vi "S_absolu.vi"(10 "Th  (Seebeck)":u16(ring)=5 items=["B", "E", "J", "K", "R", "S", "T", "N"], 11 "T, in  Kelvin":dbl) -> (1 "TC signal /microVperK":dbl, 2 "S of - wire /microV/K":dbl, 3 "S of + wire /microV/K":dbl)   [LabVIEW 2018]
panel:
  in  "error in":errorcluster
  out "error out":errorcluster
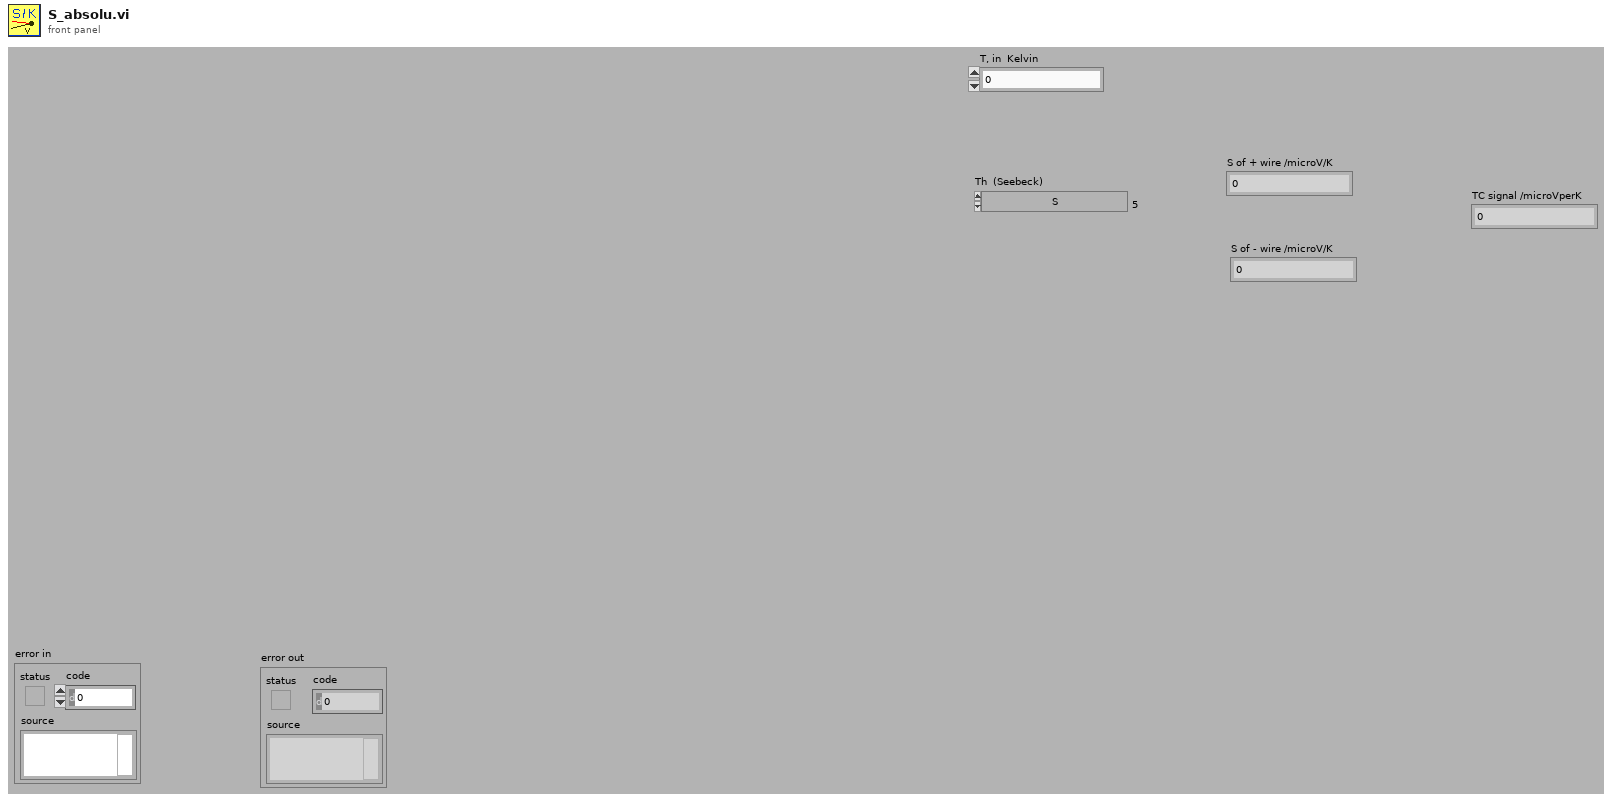
[diagram p1: front panel]
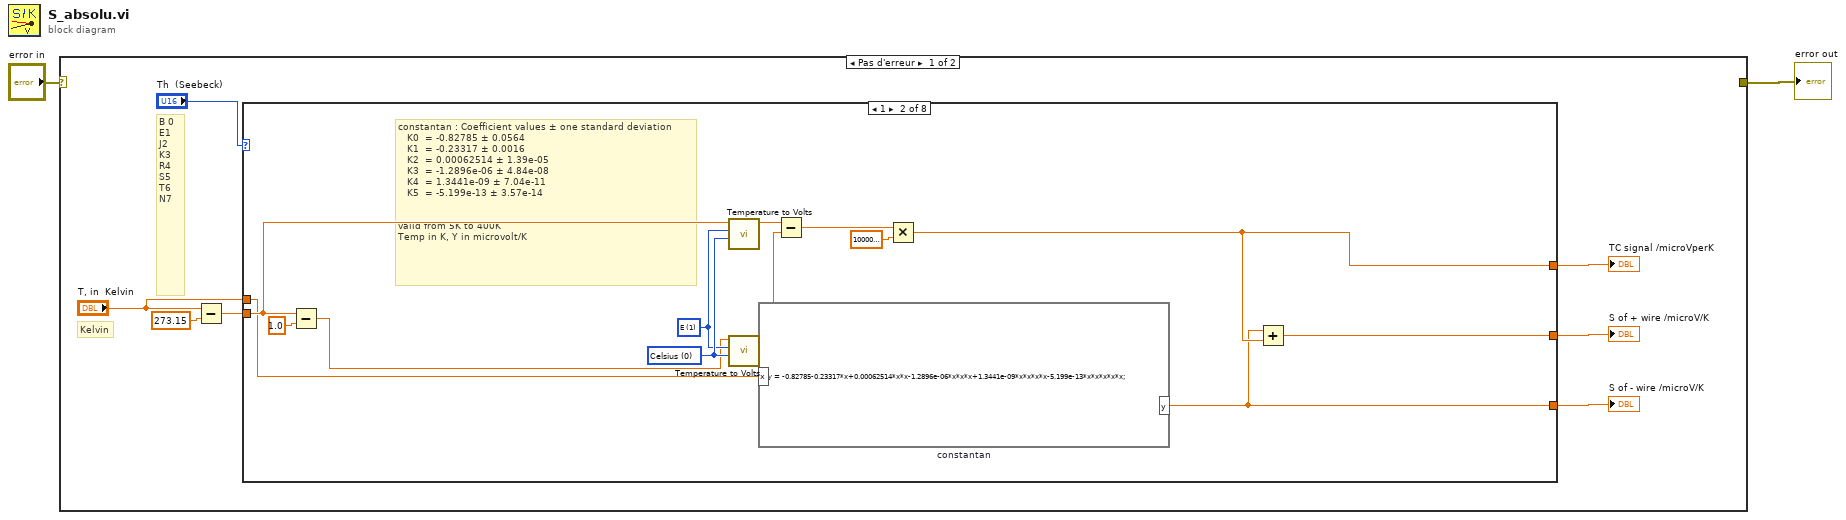
[diagram p0: block diagram]
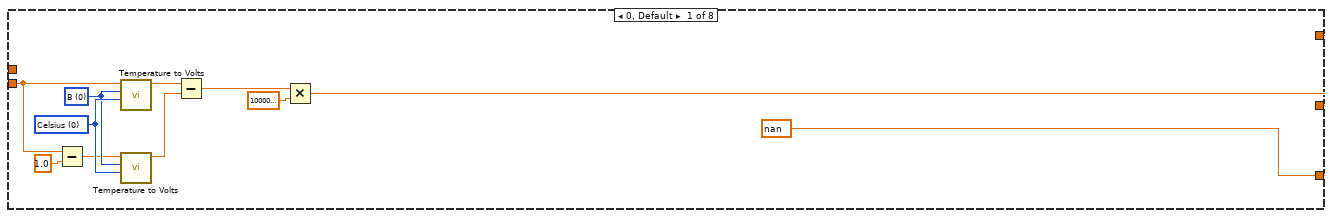
[diagram p2: hidden frame]
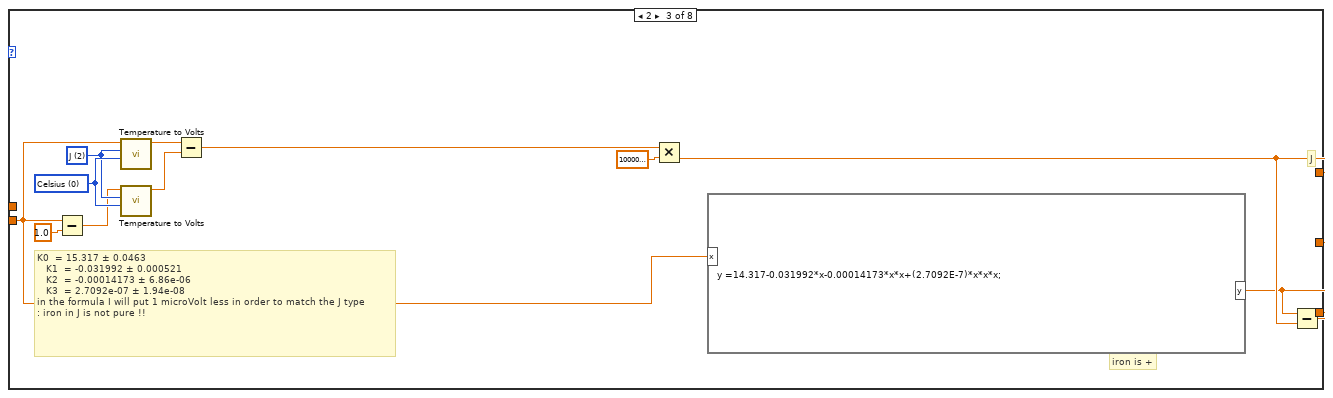
[diagram p3: hidden frame]
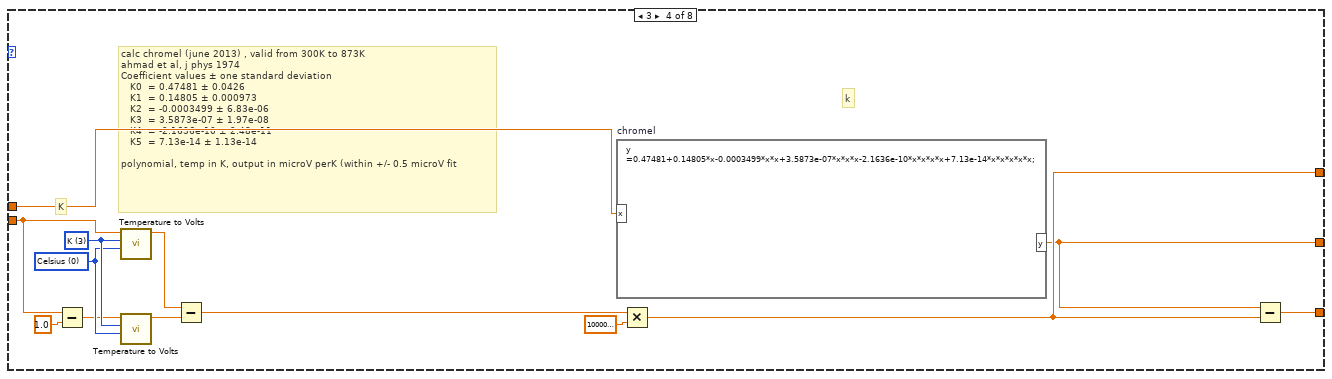
[diagram p4: hidden frame]
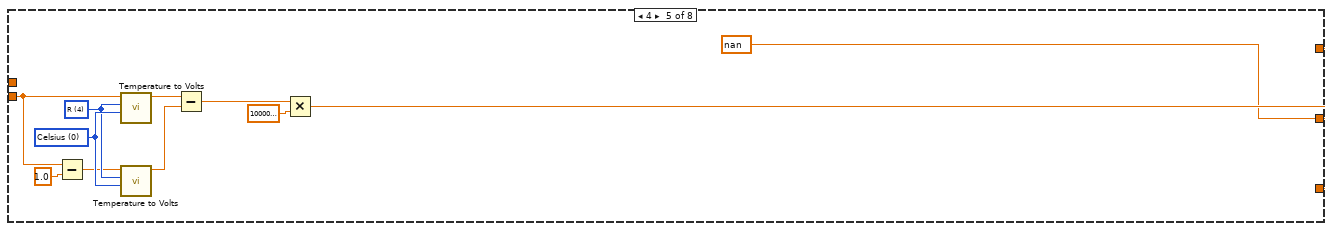
[diagram p5: hidden frame]
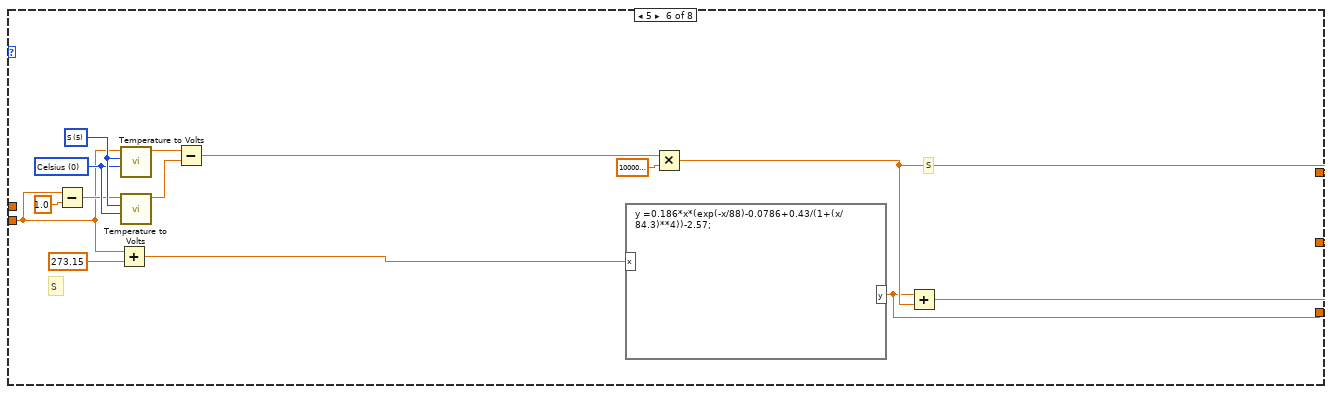
[diagram p6: hidden frame]
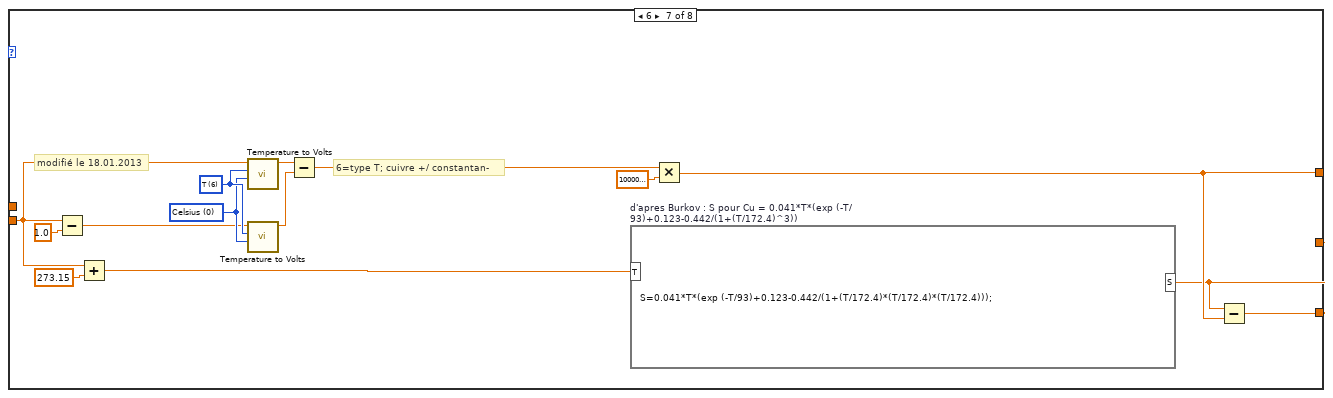
[diagram p7: hidden frame]
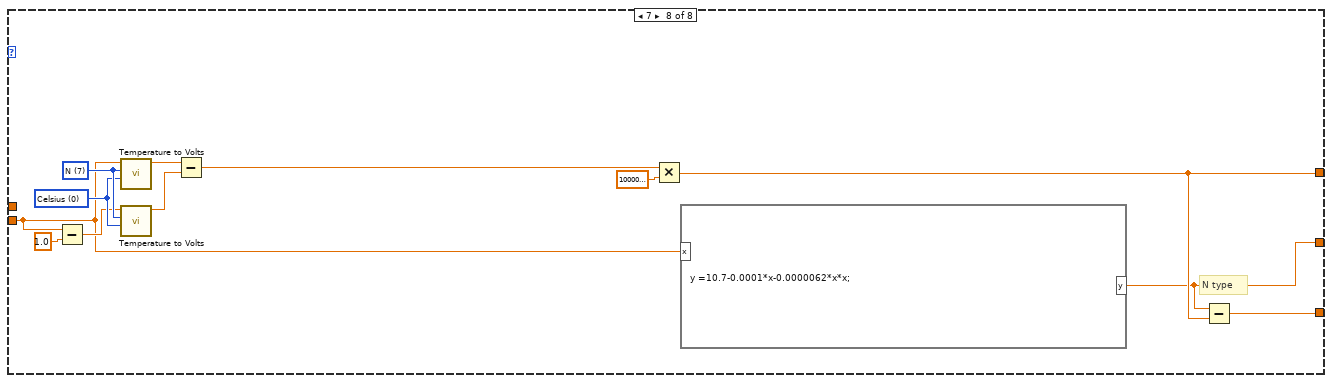
[diagram p8: hidden frame]
diagram:
  n1 = case shown="Pas d'erreur" "error in" {
    selector: "error in" -> [_ w110]
    tunnel: [_ w110] -> w2
    frame No Error {
      # "Kelvin"
      # "B 0\nE1\nJ2\nK3\nR4\nS5\nT6\nN7"
      n2 = Subtract(x="T, in  Kelvin", y=273.15) -> (x-y=w4:dbl)
      n3 = case shown="1" "Th  (Seebeck)" {
        tunnel: [w20 w22 w34 w58 w59 w70 w89 w101] -> w8
        tunnel: w4 -> [w10 w24 w37 w48 w61 w73 w85 w98]
        tunnel: [w20 w21 w35 w47 w59 w75 w84 w99] -> w6
        tunnel: [w11 w25 w36 w49 w60 w74 w88 w100] -> w7
        tunnel: "T, in  Kelvin" -> [_ w23 _ w46 _ _ _ _]
        frame 0, Default {
          w17 = u16 0 items=["B", "E", "J", "K", "R", "S", "T", "N"] ("ThermocoupleType")
          w19 = u16 0 items=["Celsius", "Fahrenheit", "Kelvin", "Rankine"] ("Temperature Units")
          w20 = nan
          n4 = Subtract(x=w10, y=1.0) -> (x-y=w15:dbl)
          n5 = call <vilib>:"Temperature to Volts.vi"("Temperature Units"=w19, "ThermocoupleType"=w17, "Temperature"=w10) -> ("Thermocouple Voltage"=w14:sgl)  [unwired: 4 out]
          n6 = call <vilib>:"Temperature to Volts.vi"("Temperature Units"=w19, "ThermocoupleType"=w17, "Temperature"=w15) -> ("Thermocouple Voltage"=w13:sgl)  [unwired: 4 out]
          n7 = Subtract(x=w14, y=w13) -> (x-y=w12:sgl)
          n8 = Multiply(x=w12, y=1000000.0) -> (x*y=w11:dbl)
        }
        frame 1 {
          w31 = u16 1 items=["B", "E", "J", "K", "R", "S", "T", "N"] ("ThermocoupleType")
          w33 = u16 0 items=["Celsius", "Fahrenheit", "Kelvin", "Rankine"] ("Temperature Units")
          # "constantan : Coefficient values ± one standard deviation\n  \tK0 \t= -0.82785 ± 0.0564\n  \tK1 \t= -0.23317 ± 0.0016\n  \tK2 \t= 0.00062514 ± 1.39e-05\n  \tK3 \t= -1.2896e-06 ± 4.84e-08\n  \tK4 \t= 1.3441e-09 ± 7.04e-11\n  \tK5 \t= -5.199e-13 ± 3.57e-14\n\n\nvalid from 5K to 400K\nTemp in K, Y in microvolt/K"
          n9 = Subtract(x=w24, y=1.0) -> (x-y=w29:dbl)
          n10 = call <vilib>:"Temperature to Volts.vi"("Temperature Units"=w33, "ThermocoupleType"=w31, "Temperature"=w24) -> ("Thermocouple Voltage"=w28:sgl)  [unwired: 4 out]
          n11 = call <vilib>:"Temperature to Volts.vi"("Temperature Units"=w33, "ThermocoupleType"=w31, "Temperature"=w29) -> ("Thermocouple Voltage"=w27:sgl)  [unwired: 4 out]
          n12 = formula code="y = -0.82785-0.23317*x+0.00062514*x*x-1.2896e-06*x*x*x+1.3441e-09*x*x*x*x-5.199e-13*x*x*x*x*x;" "constantan"("x"=w23) -> ("y"=w22:dbl)
          n13 = Subtract(x=w28, y=w27) -> (x-y=w26:sgl)
          n14 = Multiply(x=w26, y=1000000.0) -> (x*y=w25:dbl)
          n15 = Add(x=w22, y=w25) -> (x+y=w21:dbl)
        }
        frame 2 {
          w43 = u16 2 items=["B", "E", "J", "K", "R", "S", "T", "N"] ("ThermocoupleType")
          w45 = u16 0 items=["Celsius", "Fahrenheit", "Kelvin", "Rankine"] ("Temperature Units")
          # "K0 \t= 15.317 ± 0.0463\n  \tK1 \t= -0.031992 ± 0.000521\n  \tK2 \t= -0.00014173 ± 6.86e-06\n  \tK3 \t= 2.7092e-07 ± 1.94e-08\nin the formula I will put 1 microVolt less in order to match the J type\n: iron in J is not pure !!"
          # "iron is +"
          # "J"
          n16 = Subtract(x=w37, y=1.0) -> (x-y=w41:dbl)
          n17 = call <vilib>:"Temperature to Volts.vi"("Temperature Units"=w45, "ThermocoupleType"=w43, "Temperature"=w37) -> ("Thermocouple Voltage"=w40:sgl)  [unwired: 4 out]
          n18 = call <vilib>:"Temperature to Volts.vi"("Temperature Units"=w45, "ThermocoupleType"=w43, "Temperature"=w41) -> ("Thermocouple Voltage"=w39:sgl)  [unwired: 4 out]
          n19 = Subtract(x=w40, y=w39) -> (x-y=w38:sgl)
          n20 = Multiply(x=w38, y=1000000.0) -> (x*y=w36:dbl)
          n21 = formula code="y =14.317-0.031992*x-0.00014173*x*x+(2.7092E-7)*x*x*x;"("x"=w37) -> ("y"=w35:dbl)
          n22 = Subtract(x=w35, y=w36) -> (x-y=w34:dbl)
        }
        frame 3 {
          w56 = u16 3 items=["B", "E", "J", "K", "R", "S", "T", "N"] ("ThermocoupleType")
          w55 = u16 0 items=["Celsius", "Fahrenheit", "Kelvin", "Rankine"] ("Temperature Units")
          # "calc chromel (june 2013) , valid from 300K to 873K\nahmad et al, j phys 1974\nCoefficient values ± one standard deviation\n  \tK0 \t= 0.47481 ± 0.0426\n  \tK1 \t= 0.14805 ± 0.000973\n  \tK2 \t= -0.0003499 ± 6.83e-06\n  \tK3 \t= 3.5873e-07 ± 1.97e-08\n  \tK4 \t= -2.1636e-10 ± 2.48e-11\n  \tK5 \t= 7.13e-14 ± 1.13e-14\n\npolynomial, temp in K, output in microV perK (within +/- 0.5 microV fit"
          # "K"
          # "k"
          n23 = Subtract(x=w48, y=1.0) -> (x-y=w53:dbl)
          n24 = call <vilib>:"Temperature to Volts.vi"("Temperature Units"=w55, "ThermocoupleType"=w56, "Temperature"=w48) -> ("Thermocouple Voltage"=w52:sgl)  [unwired: 4 out]
          n25 = call <vilib>:"Temperature to Volts.vi"("Temperature Units"=w55, "ThermocoupleType"=w56, "Temperature"=w53) -> ("Thermocouple Voltage"=w51:sgl)  [unwired: 4 out]
          n26 = Subtract(x=w52, y=w51) -> (x-y=w50:sgl)
          n27 = formula code="y =0.47481+0.14805*x-0.0003499*x*x+3.5873e-07*x*x*x-2.1636e-10*x*x*x*x+7.13e-14*x*x*x*x*x;" "chromel"("x"=w46) -> ("y"=w47:dbl)
          n28 = Multiply(x=w50, y=1000000.0) -> (x*y=w49:dbl)
          n29 = Subtract(x=w47, y=w49) -> (x-y=w58:dbl)
        }
        frame 4 {
          w59 = nan
          w67 = u16 4 items=["B", "E", "J", "K", "R", "S", "T", "N"] ("ThermocoupleType")
          w69 = u16 0 items=["Celsius", "Fahrenheit", "Kelvin", "Rankine"] ("Temperature Units")
          n30 = Subtract(x=w61, y=1.0) -> (x-y=w65:dbl)
          n31 = call <vilib>:"Temperature to Volts.vi"("Temperature Units"=w69, "ThermocoupleType"=w67, "Temperature"=w61) -> ("Thermocouple Voltage"=w64:sgl)  [unwired: 4 out]
          n32 = call <vilib>:"Temperature to Volts.vi"("Temperature Units"=w69, "ThermocoupleType"=w67, "Temperature"=w65) -> ("Thermocouple Voltage"=w63:sgl)  [unwired: 4 out]
          n33 = Subtract(x=w64, y=w63) -> (x-y=w62:sgl)
          n34 = Multiply(x=w62, y=1000000.0) -> (x*y=w60:dbl)
        }
        frame 5 {
          w82 = u16 5 items=["B", "E", "J", "K", "R", "S", "T", "N"] ("ThermocoupleType")
          w81 = u16 0 items=["Celsius", "Fahrenheit", "Kelvin", "Rankine"] ("Temperature Units")
          # "S"
          # "S"
          n35 = Subtract(x=w73, y=1.0) -> (x-y=w79:dbl)
          n36 = Add(x=w73, y=273.15) -> (x+y=w71:dbl)
          n37 = call <vilib>:"Temperature to Volts.vi"("Temperature Units"=w81, "ThermocoupleType"=w82, "Temperature"=w73) -> ("Thermocouple Voltage"=w78:sgl)  [unwired: 4 out]
          n38 = call <vilib>:"Temperature to Volts.vi"("Temperature Units"=w81, "ThermocoupleType"=w82, "Temperature"=w79) -> ("Thermocouple Voltage"=w77:sgl)  [unwired: 4 out]
          n39 = Subtract(x=w78, y=w77) -> (x-y=w76:sgl)
          n40 = formula code="y =0.186*x*(exp(-x/88)-0.0786+0.43/(1+(x/84.3)**4))-2.57;"("x"=w71) -> ("y"=w70:dbl)
          n41 = Multiply(x=w76, y=1000000.0) -> (x*y=w74:dbl)
          n42 = Add(x=w70, y=w74) -> (x+y=w75:dbl)
        }
        frame 6 {
          w96 = u16 6 items=["B", "E", "J", "K", "R", "S", "T", "N"] ("ThermocoupleType")
          w95 = u16 0 items=["Celsius", "Fahrenheit", "Kelvin", "Rankine"] ("Temperature Units")
          # "6=type T; cuivre +/ constantan-"
          # "modifié le 18.01.2013"
          n43 = Subtract(x=w85, y=1.0) -> (x-y=w93:dbl)
          n44 = Add(x=w85, y=273.15 ("T in C")) -> (x+y=w87:dbl)
          n45 = call <vilib>:"Temperature to Volts.vi"("Temperature Units"=w95, "ThermocoupleType"=w96, "Temperature"=w85) -> ("Thermocouple Voltage"=w92:sgl)  [unwired: 4 out]
          n46 = call <vilib>:"Temperature to Volts.vi"("Temperature Units"=w95, "ThermocoupleType"=w96, "Temperature"=w93) -> ("Thermocouple Voltage"=w91:sgl)  [unwired: 4 out]
          n47 = Subtract(x=w92, y=w91) -> (x-y=w90:sgl)
          n48 = formula code="S=0.041*T*(exp (-T/93)+0.123-0.442/(1+(T/172.4)*(T/172.4)*(T/172.4)));" "d'apres Burkov : S pour Cu = 0.041*T*(exp (-T/93)+0.123-0.442/(1+(T/172.4)^3))"("T"=w87) -> ("S"=w84:dbl)
          n49 = Multiply(x=w90, y=1000000.0) -> (x*y=w88:dbl)
          n50 = Subtract(x=w84, y=w88) -> (x-y=w89:dbl)
        }
        frame 7 {
          w108 = u16 7 items=["B", "E", "J", "K", "R", "S", "T", "N"] ("ThermocoupleType")
          w107 = u16 0 items=["Celsius", "Fahrenheit", "Kelvin", "Rankine"] ("Temperature Units")
          # "N type"
          n51 = Subtract(x=w98, y=1.0) -> (x-y=w105:dbl)
          n52 = call <vilib>:"Temperature to Volts.vi"("Temperature Units"=w107, "ThermocoupleType"=w108, "Temperature"=w98) -> ("Thermocouple Voltage"=w104:sgl)  [unwired: 4 out]
          n53 = call <vilib>:"Temperature to Volts.vi"("Temperature Units"=w107, "ThermocoupleType"=w108, "Temperature"=w105) -> ("Thermocouple Voltage"=w103:sgl)  [unwired: 4 out]
          n54 = Subtract(x=w104, y=w103) -> (x-y=w102:sgl)
          n55 = Multiply(x=w102, y=1000000.0) -> (x*y=w100:dbl)
          n56 = formula code="y =10.7-0.0001*x-0.0000062*x*x;"("x"=w98) -> ("y"=w99:dbl)
          n57 = Subtract(x=w99, y=w100) -> (x-y=w101:dbl)
        }
      }
      "S of - wire /microV/K" <- w8
      "S of + wire /microV/K" <- w6
      "TC signal /microVperK" <- w7
    }
    frame Error {
    }
  }
  "error out" <- w2
